vi "Revision Query.vi"(8 "error in (no error)":errorcluster, 11 "VISA resource name":refnum<visa-resource-name>) -> (0 "error out":errorcluster, 1 "Instrument Firmware Revision":string, 2 "Instrument Driver Revision":string, 3 "VISA resource name out":refnum<visa-resource-name>)   [LabVIEW 2017, in "Andeen-Hagerling 2700.lvlib"]
doc: "Queries the current instrument firmware revision and instrument driver revision.\n\nRefer to the Readme file for detailed driver information including modification history."
uses:
  Andeen-Hagerling 2700.lvlib
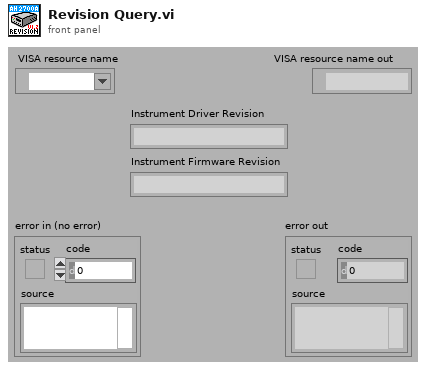
[diagram p1: front panel]
types:
  T1 = enum32{"invalid app kind", "Development System", "Run Time System", "Student Edition", "Embedded LabVIEW", "Evaluation", "Custom"}
  T2 = cluster{"Major":u16, "Minor":u16, "Fix":u16, "Build":u16}
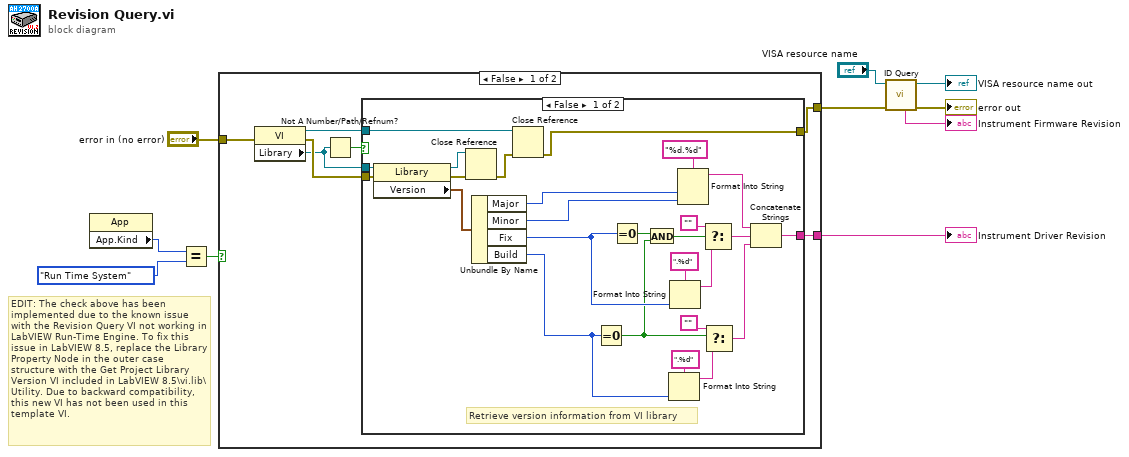
[diagram p0: block diagram]
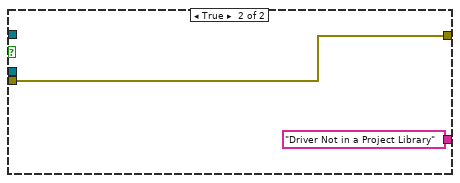
[diagram p2: hidden frame]
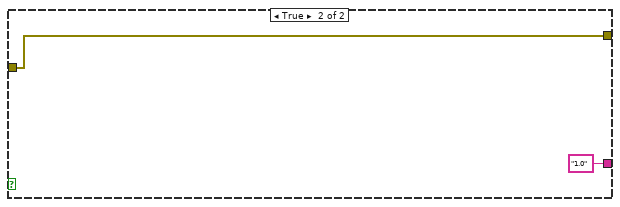
[diagram p3: hidden frame]
diagram:
  # "EDIT: The check above has been implemented due to the known issue with the Revision Query VI not working in LabVIEW Run-Time Engine. To fix this issue in LabVIEW 8.5, replace the Library Property Node in the outer case structure with the Get Project Library Version VI included in LabVIEW 8.5\\vi.lib\\Utility. Due to backward compatibility, this new VI has not been used in this template VI."
  n1 = property class="App"() -> ("App.Kind"=w7:T1)  [unwired: 2 in, 2 out]
  n2 = Equal?(x=w7, y=T1."Run Time System" ("Application:Kind")) -> (x = y?=w8:bool)
  n3 = case shown="False" w8 {
    tunnel: [w13 "1.0"] -> w10
    tunnel: "error in (no error)" -> [w12 w46]
    tunnel: [w11 w46] -> w4
    frame False {
      n4 = property class="VI"(error in=w12) -> (reference out=w17:refnum<vi>, error out=w16:errorcluster, "Library"=w15:refnum<vi>)  [unwired: 1 in]
      n5 = Not A Number/Path/Refnum?(number/path/refnum=w15) -> (NaN/Path/Refnum?=w14:bool)
      n6 = case shown="False" w14 {
        tunnel: w17 -> [w40 _]
        tunnel: w16 -> [w25 w45]
        tunnel: [w20 w45] -> w11
        tunnel: [w19 "Driver Not in a Project Library"] -> w13
        tunnel: w15 -> [w18 _]
        frame False {
          # "Retrieve version information from VI library"
          n7 = property class="Library"(reference=w18, error in=w25) -> (reference out=w42:refnum<vi>, error out=w43:errorcluster, "Version"=w39:T2)
          n8 = Close Reference(reference=w42, error in (no error)=w43) -> (error out=w41:errorcluster)
          n9 = Unbundle By Name(w39) -> ("Major"=w28:u16, "Minor"=w27:u16, "Fix"=w24:u16, "Build"=w26:u16)
          n10 = Close Reference(reference=w40, error in (no error)=w41) -> (error out=w20:errorcluster)
          n11 = Equal To 0?(x=w26) -> (x = 0?=w22:bool)
          n12 = Equal To 0?(x=w24) -> (x = 0?=w23:bool)
          n13 = And(x=w23, y=w22) -> (x .and. y?=w21:bool)
          n14 = Format Into String(format string=".%d", w26) -> (resulting string=w32:string)  [unwired: 2 in, 1 out]
          n15 = Format Into String(format string=".%d", w24) -> (resulting string=w36:string)  [unwired: 2 in, 1 out]
          n16 = Format Into String(format string="%d.%d", w28, w27) -> (resulting string=w34:string)  [unwired: 2 in, 1 out]
          n17 = Select(t="", s=w21, f=w36) -> (s? t:f=w33:string)
          n18 = Select(t="", s=w22, f=w32) -> (s? t:f=w29:string)
          n19 = Concatenate Strings(w34, w33, w29) -> (w19:string)
        }
        frame True {
        }
      }
    }
    frame True {
    }
  }
  "Instrument Driver Revision" <- w10
  n20 = call "ID Query.vi"("error in"=w4, "VISA resource name"="VISA resource name") -> ("error out"=→"error out":errorcluster, "VISA resource name out"=→"VISA resource name out":refnum<visa-resource-name>, "Firmware Revision"=→"Instrument Firmware Revision":string)  [unwired: 4 in, 3 out]
